vi "QUBE-Servo 2 ROTPEN State Space Modeling - Impulse.vi"() -> ()   [LabVIEW 2016]
uses:
  <vilib>/Simulation/Scripting/Companion Diagram/SimConfigNode/SimParams.ctl
  <vilib>/Simulation/Scripting/Companion Diagram/SimConfigNode/_simSolvers.ctl
  <vilib>/Simulation/Implementation/Shared/SIMSCR Execution Mode.ctl
  <vilib>/Platform/TimedLoop/XDataNode/timing_clust.ctl
  <vilib>/Platform/TimedLoop/XDataNode/nitl_modes.ctl
  <vilib>/Platform/TimedLoop/XDataNode/wakeup.ctl
  <vilib>/Simulation/Param Hierarchy/Typedefs/SIMPH Param Control Actions.ctl
  <vilib>/Simulation/Implementation/Shared/NILVSim_ParamChanged.vi
  <vilib>/Simulation/Implementation/Shared/NILVSim_FinishedLate.vi
  <vilib>/Simulation/Implementation/Shared/NILVSIM_BeginStep.vi
  <vilib>/Simulation/DataSources/Implementation/NILVSim Pulse Generator.llb/SIM Pulse Generator (scalar).vi
  <vilib>/Simulation/SignalArithmetic/Implementation/NILVSim Gain.llb/SIM Gain (scalar).vi
  <vilib>/Simulation/Utility/Implementation/SIM Halt.vi
  <vilib>/Simulation/ContinuousLinear/Implementation/NILVSim State Space.llb/SIM State Space Distributor (CD).vi
  <vilib>/Simulation/ContinuousLinear/Implementation/NILVSim State Space.llb/SIM State Space Collector (CD).vi
  <vilib>/Simulation/Implementation/Shared/NILVSim_Manager.vi
  <vilib>/Utility/error.llb/Clear Errors.vi
  <vilib>/Simulation/Implementation/Shared/NILVSim_FinalizeModel.vi
  <vilib>/imath/engines/lvmath2/RunTimeEngine/IndexRead/NIMS M(S,S).vi
  <instcachedir>/0/NIMS M(S,S)_AC51E74150A542F7991B9634C66F3096.lvgen/NIMS M(S,S)_AC51E74150A542F7991B9634C66F3096_002.vi
  <vilib>/imath/engines/lvmath2/RunTimeEngine/IndexRead/NIMS V(S).vi
  <instcachedir>/0/NIMS V(S)_0488751826AF41519A22953C041130DC.lvgen/NIMS V(S)_0488751826AF41519A22953C041130DC_000.vi
  <vilib>/imath/engines/lvmath2/RunTimeEngine/IndexReplace/NIMS M(S,S)=S.vi
  <instcachedir>/0/NIMS M(S,S)=S_98E40400474E4398B113AE20298B4F82.lvgen/NIMS M(S,S)=S_98E40400474E4398B113AE20298B4F82_000.vi
  <vilib>/imath/engines/lvmath2/RunTimeEngine/ErrorHandling/NIMS_Create Error From Enums.vi
  <instcachedir>/0/NIMS M(S,S)_AC51E74150A542F7991B9634C66F3096.lvgen/NIMS M(S,S)_AC51E74150A542F7991B9634C66F3096_000.vi
  <vilib>/imath/engines/lvmath/Plug In/Control Design/BuiltInFunctions/ss/NIMS_CD_ss(A,B,C,D).vi
  <vilib>/imath/engines/lvmath2/RunTimeEngine/NodeEndStatement/NIMS_NodeEndStatement_Output.vi
  <instcachedir>/0/NIMS_NodeEndStatement_Output_53EC0D466D134D7ABD903AC30B43404B.lvgen/NIMS_NodeEndStatement_Output_53EC0D466D134D7ABD903AC30B43404B_010.vi
  <vilib>/imath/engines/lvmath2/RunTimeEngine/ErrorHandling/NIMS_Finalize Error.vi
  <vilib>/Simulation/Implementation/Shared/SIM Unbundle Sim Info.vi
  <vilib>/Simulation/Implementation/Shared/SIMSH Read Queue.vi
  <vilib>/Simulation/Implementation/Shared/NILVSim_Initialize.vi
  <vilib>/Simulation/Utility/Implementation/NILVSim Get Time and IsAcceptedStep.vi
  SubVIs/QUBE2 RW.vi
  <vilib>/Simulation/Implementation/Shared/NILVSim_GetModelError.vi
  <vilib>/Simulation/Implementation/Shared/SIM Bundle Sim Info.vi
  <vilib>/addons/Control Design/_Utility/Model Viewer.llb/Model Viewer SubVI/cd_Draw State-Space Equation (SS).vi
  <vilib>/Simulation/Scripting/Companion Diagram/SimConfigNode/SimDog.xnode
  <vilib>/addons/Control Design/_Model Construction/Model Typedefs.llb/CD State Space Model (MIMO).ctl
  <vilib>/addons/Control Design/_Model Construction/Model Typedefs.llb/CD General Elements.ctl
  <vilib>/Platform/TimedLoop/XDataNode/XDataNode.xnode
  <vilib>/Simulation/Implementation/XNodeFramework/SimXNode/SimX.xnode
  <vilib>/addons/Control Design/_Model Construction/NI_LinSys_Model Typedefs.lvlib
  <vilib>/addons/Control Design/_Utility/NI_CD_Model Viewer.lvlib
  <vilib>/Simulation/ContinuousLinear/Implementation/NILVSim State Space.llb/SIM State Space (CD).vi
  <vilib>/Platform/TimedLoop/XDataNode/XDNodeRunTimeDep.lvlib
  <vilib>/Simulation/Implementation/Shared/NI_SIM_Implementation.lvlib
panel:
  out "Stall Error":bool
  out "Open Loop State-Space Model":picture
  out "Error":errorcluster
  in  "Stop Button":bool
  in  "Motor Parameters":T1={"Rm (ohm)"=8.4, "km (V-s/rad)"=0.042, "kt (N-m/A)"=0.042} {"kt (N-m/A)" min=0.0 format="%_3g"; "km (V-s/rad)" min=0.0 format="%_3g"; "Rm (ohm)" min=0.0 format="%_3f"}
  in  "Pendulum Parameters":T2={"Mp (kg)"=0.024, "Lr (m)"=0.085, "Lp (m)"=0.129, "Jr (kg.m^2)"=5.72e-05, "Dr (N.m.s/rad)"=0.0015, "Jp (kg.m^2)"=3.33e-05, "Dp (N.m.s/rad)"=0.0005, "g (m/s^2)"=9.81} {"g (m/s^2)" min=0.0 format="%_3g"; "Lr (m)" min=0.0 format="%_3g"; "Dr (N.m.s/rad)" min=0.0 format="%_3g"; "Jr (kg.m^2)" min=0.0 format="%_3g"; "Dp (N.m.s/rad)" min=0.0 format="%_3g"; "Jp (kg.m^2)" min=0.0 format="%_3g"; "Lp (m)" min=0.0 format="%_3g"; "Mp (kg)" min=0.0 format="%_3f"}
  out "Pendulum Angle (rad)":cluster{"output":dbl, dbl}(graph)
  out "Rotary Arm Angle (rad)":cluster{"output":dbl, dbl}(graph)
  # "Rotary Motion Platform"
  # "QUBE-Servo 2 | State Space Modeling (Impulse Response)"
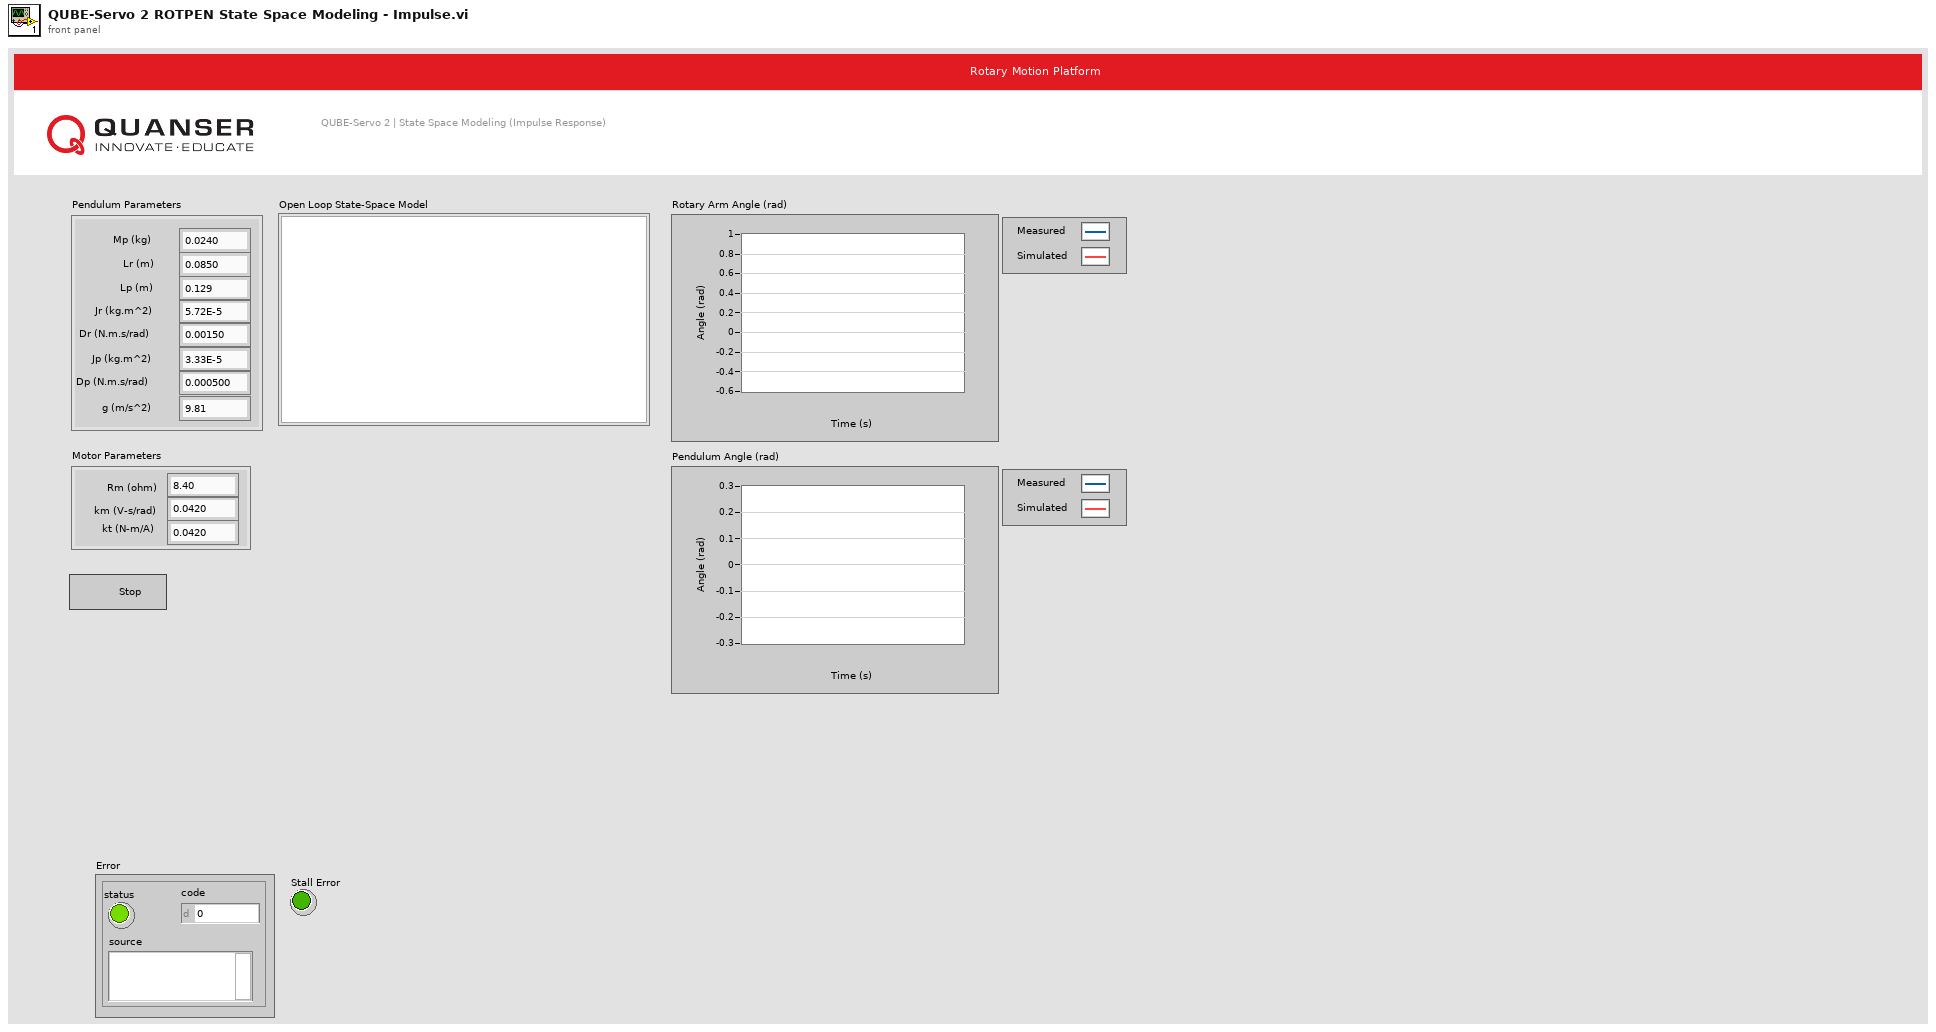
[diagram p1: front panel]
types:
  T1 = cluster{"Rm (ohm)":dbl, "km (V-s/rad)":dbl, "kt (N-m/A)":dbl}
  T2 = cluster{"Mp (kg)":dbl, "Lr (m)":dbl, "Lp (m)":dbl, "Jr (kg.m^2)":dbl, "Dr (N.m.s/rad)":dbl, "Jp (kg.m^2)":dbl, "Dp (N.m.s/rad)":dbl, "g (m/s^2)":dbl}
  T3 = typedef "QFLEX myRIO.ctl" = cluster{"Error":errorcluster, "CS DO Ref":T4, "SPI Ref":T11}
  T4 = typedef "DIO.lvlib/DIO Reference.ctl" = cluster{"myRIO Reference":T5, "DIO Channels List":T9}
  T5 = typedef "myRIO Generic Hardware Reference.ctl" = cluster{"myRIO Model":T6, "myRIO Hardware Reference":T7}
  T6 = typedef "Hardware Version Enum.ctl" = enum16{"Unknown", "myRIO-1900", "myRIO-1950", "roboRIO", "NI ELVIS RIO CM"}
  T7 = typedef "myRIO v1.0 Reference.ctl" = cluster{"Generic FPGA Reference":T8, "Allow multiple opens":bool}
  T8 = typedef "Generic FPGA Reference.ctl" = refnum<k20>
  T9 = typedef "DIO Channels List.ctl" = T10[]
  T10 = typedef "DIO Channels Enum.ctl" = enum16{"Not Connected", "C/DIO0", "C/DIO1", "C/DIO2", "C/DIO3", "C/DIO4", "C/DIO5", "C/DIO6", "C/DIO7", "A/DIO0", "A/DIO1", "A/DIO2", "A/DIO3", "A/DIO4", "A/DIO5", "A/DIO6", "A/DIO7", "A/DIO8", "A/DIO9", "A/DIO10", "A/DIO11", "A/DIO12", "A/DIO13", "A/DIO14", "A/DIO15", "B/DIO0", "B/DIO1", "B/DIO2", "B/DIO3", "B/DIO4", "B/DIO5", "B/DIO6", "B/DIO7", "B/DIO8", "B/DIO9", "B/DIO10", "B/DIO11", "B/DIO12", "B/DIO13", "B/DIO14", "B/DIO15", "LED0", "LED1", "LED2", "LED3", "Button0", "DIO/DIO0", "DIO/DIO1", "DIO/DIO2", "DIO/DIO3", "DIO/DIO4", "DIO/DIO5", "DIO/DIO6", "DIO/DIO7", "DIO/DIO8", "DIO/DIO9", "SPI/CS0", "SPI/CS1", "SPI/CS2", "SPI/CS3", "LED RADIO (Green)", "LED RADIO (Red)", "LED COMM (Green)", "LED COMM (Red)", "LED MODE (Green)", "LED MODE (Red)"}
  T11 = typedef "SPI.lvlib/SPI Reference.ctl" = cluster{"myRIO Reference":T5, "SPI Channels Enum":T12, "SPI Configuration":T13}
  T12 = typedef "SPI Channels Enum.ctl" = enum16{"Not Connected", "A/SPI", "B/SPI", "SPI/SPI"}
  T13 = typedef "SPI.lvlib/SPI Configuration.ctl" = cluster{"Frequency [Hz]":dbl, "Clock Phase":T14, "Clock Polarity":T15, "Data Direction":T16, "Frame Length":T17}
  T14 = typedef "SPI Clock Phase.ctl" = enum8{"Leading", "Trailing"}
  T15 = typedef "SPI Clock Polarity.ctl" = enum8{"Low", "High"}
  T16 = typedef "SPI Data Direction.ctl" = enum8{"Most significant bit first", "Least significant bit first"}
  T17 = typedef "SPI Frame Length.ctl" = u8
  T18 = typedef "NI_LinSys_Model Typedefs.lvlib/CD State Space Model (MIMO).ctl" = cluster{"properties":T19, "A":dbl[][], "B":dbl[][], "C":dbl[][], "D":dbl[][], "StateNames":string[], "Transport Delay":dbl[][]}
  T19 = typedef "NI_LinSys_Model Typedefs.lvlib/CD General Elements.ctl" = cluster{"Model name":string, "Input names":string[], "Output names":string[], "Input Delays":dbl[], "Output Delays":dbl[], "Sampling Time":dbl, "Notes":string}
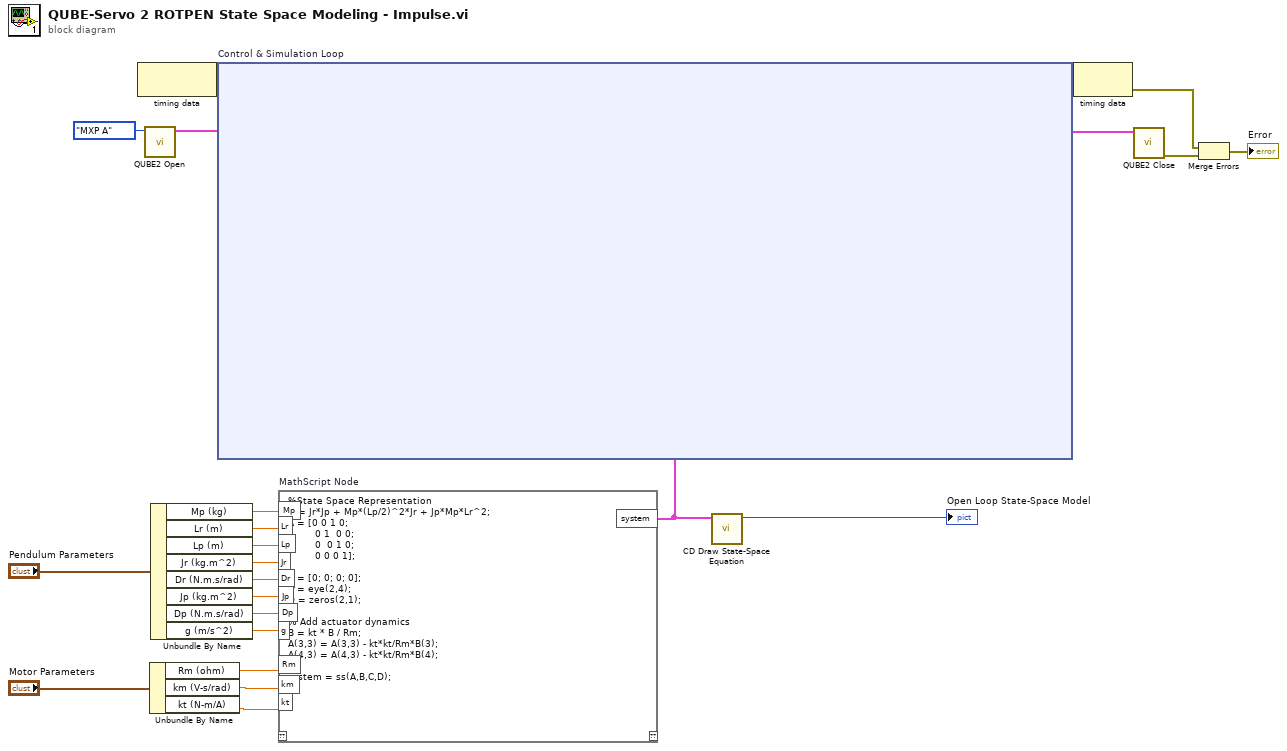
[diagram p0: block diagram]
diagram:
  n1 = node-c288() -> (w23:variant)  [unwired: 1 in]
  n2 = call "QUBE2 Open.vi"("Connector"=enum16{"MXP A", "MXP B"}."MXP A") -> ("QFLEX Cluster Out"=w4:T3)  [unwired: 10 in]
  n3 = Unbundle By Name ("Unbundle By Name 2")("Motor Parameters") -> ("Rm (ohm)"=w13:dbl, "km (V-s/rad)"=w12:dbl, "kt (N-m/A)"=w11:dbl)
  n4 = Unbundle By Name("Pendulum Parameters") -> ("Mp (kg)"=w21:dbl, "Lr (m)"=w20:dbl, "Lp (m)"=w19:dbl, "Jr (kg.m^2)"=w18:dbl, "Dr (N.m.s/rad)"=w17:dbl, "Jp (kg.m^2)"=w16:dbl, "Dp (N.m.s/rad)"=w15:dbl, "g (m/s^2)"=w14:dbl)
  n5 = mathscript code="%State Space Representation\nJt = Jr*Jp + Mp*(Lp/2)^2*Jr + Jp*Mp*Lr^2;\nA = [0 0 1 0;\n         0 1  0 0;\n         0  0 1 0;\n         0 0 0 1];\n\nB = [0; 0; 0; 0];\nC = eye(2,4);\nD = zeros(2,1);\n\n% Add actuator dynamics\nB = kt * B / Rm;\nA(3,3) = A(3,3) - kt*kt/Rm*B(3);\nA(4,3) = A(4,3) - kt*kt/Rm*B(4);\n\nsystem = ss(A,B,C,D);"("Mp"=w21, "Lr"=w20, "Lp"=w19, "Jr"=w18, "Dr"=w17, "Jp"=w16, "Dp"=w15, "g"=w14, "kt"=w11, "km"=w12, "Rm"=w13) -> ("system"=w8:T18)  [unwired: 1 in, 1 out]
  n6 = node-c254 "Control & Simulation Loop"(w23, w8, w4) -> (w22:variant, w3:T3)
  n7 = call-poly <vilib>:"CD Draw State-Space Equation.vi"("State-Space Model"=w8) -> ("Equation"=→"Open Loop State-Space Model":picture)  [unwired: 8 in, 2 out]
  n8 = node-c288(w22) -> (w1:errorcluster)
  n9 = call "QUBE2 Close.vi"("QFLEX Cluster In"=w3) -> ("error out"=w5:errorcluster)  [unwired: 10 in]
  n10 = Merge Errors(w1, w5) -> (→"Error":errorcluster)
